vi "appendTableWithCellStyles.vi"(8 "error in (no error)":errorcluster, 9 "Cell.Styles":refnum<class "Style.lvclass">[][](array[class]), 10 "Table":string[][](array[string]), 11 "xwpfTable in":refnum<class "xwpfTable.lvclass">) -> (0 "error out":errorcluster, 3 "xwpfTable out":refnum<class "xwpfTable.lvclass">)   [LabVIEW 2017, in "Word_Specific.lvlib" / "xwpfTable.lvclass"]
uses:
  xwpfTable.lvclass
  Styles/Style/Style.lvclass
  xwpfTable.lvclass/xwpfTable.ctl
  C:/Users/Neo/Desktop/Dev_Tools_BR/LabVIEW_NPOI/lib/NPOI 2.1.1/NPOI.OOXML.dll
  lib/NPOI 2.1.1/NPOI.OOXML.dll
  xwpfParagraph/xwpfParagraph.lvclass
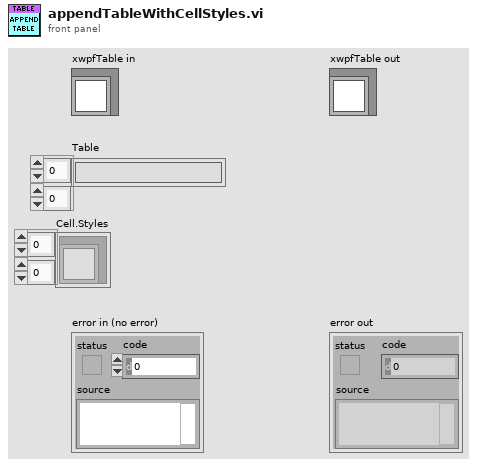
[diagram p1: front panel]
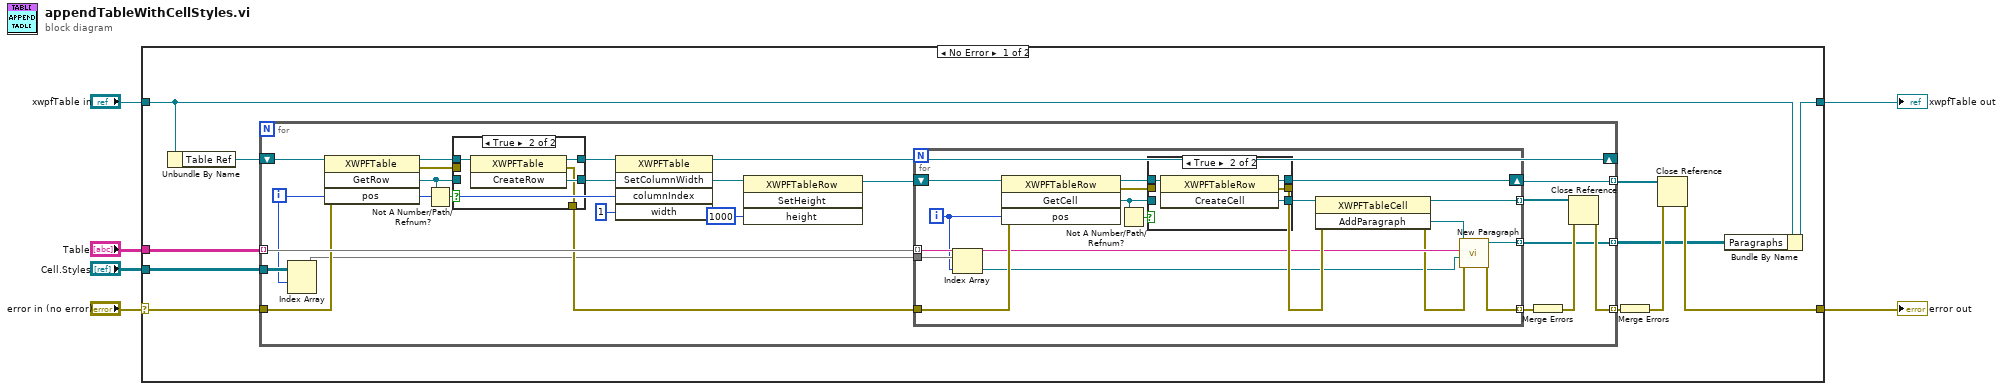
[diagram p0: block diagram]
diagram:
  n1 = case shown="No Error" "error in (no error)" {
    selector: "error in (no error)" -> [w13 w74]
    tunnel: [w12 w74] -> w5
    tunnel: [w9 w73] -> w3
    tunnel: "xwpfTable in" -> [w17 w73]
    tunnel: "Table" -> [w15 _]
    tunnel: "Cell.Styles" -> [w7 _]
    frame No Error {
      n2 = Unbundle By Name(w17) -> ("Table Ref"=w16:refnum<k24>)
      n3 = for {
        shift-right: [w25] -> _
        shift-left: w16 -> [w40]
        tunnel: w15 -> [w36] mode=indexing
        tunnel: [w35] -> w14 mode=indexing
        tunnel: [w28] -> w11 mode=indexing
        tunnel: w13 -> [w31]
        tunnel: [w27] -> w8 mode=indexing
        tunnel: w7 -> [w20]
        i -> [w19]
        n4 = Index Array(array=w20, index (row)=w19) -> (element=w18:refnum<class "Style.lvclass">[])  [unwired: 1 in]
        n5 = invoke class="XWPFTable" method="GetRow"(reference=w40, error in=w31, "pos"=w19) -> (reference out=w37:refnum<k24>, error out=w33:errorcluster, "GetRow"=w38:refnum<k24>)  [unwired: 1 in, 1 out]
        n6 = Not A Number/Path/Refnum?(number/path/refnum=w38) -> (NaN/Path/Refnum?=w39:bool)
        n7 = case shown="True" w39 {
          tunnel: w38 -> [w68 _]
          tunnel: w37 -> [w67 w72]
          tunnel: [w68 w71] -> w24
          tunnel: [w67 w70] -> w26
          tunnel: [w66 w69] -> w32
          tunnel: w33 -> [w66 _]
          frame False {
          }
          frame True {
            n8 = invoke class="XWPFTable" method="CreateRow"(reference=w72) -> (reference out=w70:refnum<k24>, error out=w69:errorcluster, "CreateRow"=w71:refnum<k24>)  [unwired: 2 in]
          }
        }
        n9 = invoke class="XWPFTable" method="SetColumnWidth"(reference=w26, "columnIndex"=w19, "width"=u64 1) -> (reference out=w25:refnum<k24>)  [unwired: 2 in, 4 out]
        n10 = invoke class="XWPFTableRow" method="SetHeight"(reference=w24, "height"=1000) -> (reference out=w23:refnum<k24>)  [unwired: 2 in, 3 out]
        n11 = for {
          shift-right: [w54] -> w35
          shift-left: w23 -> [w58]
          tunnel: w36 -> [w47] mode=indexing
          tunnel: [w52] -> w34 mode=indexing
          tunnel: [w45] -> w30 mode=indexing
          tunnel: w32 -> [w51]
          tunnel: [w44] -> w27 mode=indexing
          tunnel: w18 -> [w43]
          i -> [w42]
          n12 = Index Array(array=w43, index=w42) -> (element=w41:refnum<class "Style.lvclass">)
          n13 = invoke class="XWPFTableRow" method="GetCell"(reference=w58, error in=w51, "pos"=w42) -> (reference out=w57:refnum<k24>, error out=w50:errorcluster, "GetCell"=w56:refnum<k24>)  [unwired: 1 in, 1 out]
          n14 = Not A Number/Path/Refnum?(number/path/refnum=w56) -> (NaN/Path/Refnum?=w55:bool)
          n15 = case shown="True" w55 {
            tunnel: w56 -> [w61 _]
            tunnel: w57 -> [w60 w65]
            tunnel: [w61 w64] -> w53
            tunnel: [w60 w63] -> w54
            tunnel: w50 -> [w59 _]
            tunnel: [w59 w62] -> w49
            frame False {
            }
            frame True {
              n16 = invoke class="XWPFTableRow" method="CreateCell"(reference=w65) -> (reference out=w63:refnum<k24>, error out=w62:errorcluster, "CreateCell"=w64:refnum<k24>)  [unwired: 2 in]
            }
          }
          n17 = invoke class="XWPFTableCell" method="AddParagraph"(reference=w53, error in=w49) -> (reference out=w52:refnum<k24>, error out=w46:errorcluster, "AddParagraph"=w48:refnum<k24>)  [unwired: 1 in]
          n18 = call "New Paragraph.vi"("error in (no error)"=w46, "Paragraph.Style"=w41, "Paragraph.Text"=w47, "Paragraph.Ref"=w48) -> ("error out"=w45:errorcluster, "xwpfParagraph out"=w44:refnum<class "xwpfParagraph.lvclass">)  [unwired: 6 in]
        }
        n19 = Merge Errors(w30) -> (w29:errorcluster)
        n20 = Close Reference(reference=w34, error in (no error)=w29) -> (error out=w28:errorcluster)
      }
      n21 = Merge Errors(w11) -> (w10:errorcluster)
      n22 = Close Reference(reference=w14, error in (no error)=w10) -> (error out=w12:errorcluster)
      n23 = Bundle By Name(cluster=w17, "Paragraphs"=w8) -> (w9:refnum<class "xwpfTable.lvclass">)
    }
    frame Error {
    }
  }
  "error out" <- w5
  "xwpfTable out" <- w3
